vi "Is Command Refnum.vi"(8 "error in (no error)":errorcluster, 11 "Command/Response Refnum in":T1 format="%.0x") -> (0 "error out":errorcluster, 2 "Is Command?":bool, 3 "Command/Response out":string)   [LabVIEW 2018, in "Instrument Addon Scripting API.lvlib"]
uses:
  Instrument Addon Scripting API.lvlib
  <vilib>/NI Veristand/Custom Device API/Custom Device Item Ref.ctl
  Addon/Addon Shared/SubVIs/Constants.vi
  Addon/Addon Shared/Instrument Addon Shared.lvlib
  <vilib>/NI VeriStand/Custom Device API/Custom Device API.lvlib
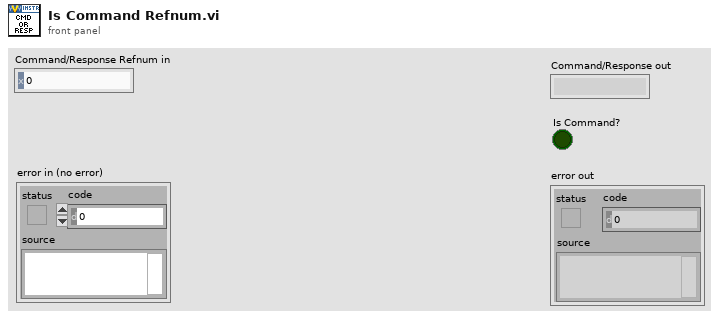
[diagram p1: front panel]
types:
  T1 = typedef "Custom Device API.lvlib/Custom Device Item Ref.ctl" = u64
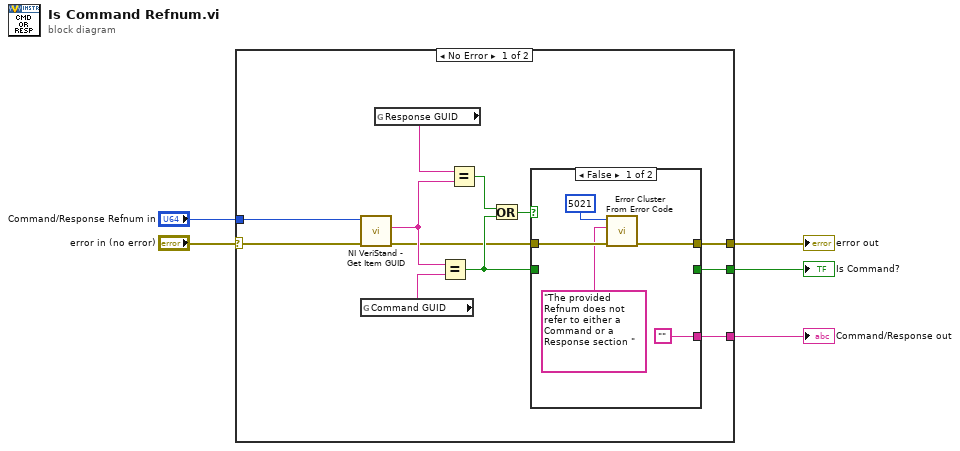
[diagram p0: block diagram]
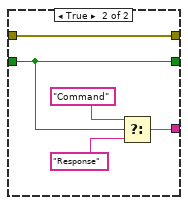
[diagram p2: hidden frame]
diagram:
  n1 = case shown="No Error" "error in (no error)" {
    selector: "error in (no error)" -> [w14 w28]
    tunnel: [w6 _] -> w5
    tunnel: [w8 w28] -> w4
    tunnel: "Command/Response Refnum in" -> [w16 _]
    tunnel: [w15 _] -> w2
    frame No Error {
      n2 = call <vilib>:"NI VeriStand - Get Item GUID.vi"("error in (no error)"=w14, "Item Ref in"=w16) -> ("error out"=w9:errorcluster, "GUID"=w12:string)  [unwired: 7 in, 1 out]
      n3 = global read "Constants.vi" "Command GUID"() -> (w17:string)
      n4 = global read "Constants.vi" "Response GUID"() -> (w13:string)
      n5 = Equal?(x=w12, y=w17) -> (x = y?=w11:bool)
      n6 = Equal?(x=w13, y=w12) -> (x = y?=w10:bool)
      n7 = Or(x=w10, y=w11) -> (x .or. y?=w7:bool)
      n8 = case shown="False" w7 {
        tunnel: ["" w25] -> w15
        tunnel: w11 -> [_ w23]
        tunnel: w9 -> [w21 w24]
        tunnel: [w20 w24] -> w8
        tunnel: [_ w23] -> w6
        frame False {
          n9 = call <vilib>:"Error Cluster From Error Code.vi"("error in (no error)"=w21, "error message (\"\")"="The provided Refnum does not refer to either a Command or a Response section " ("error message (\"\")"), "error code (0)"=5021) -> ("error out"=w20:errorcluster)  [unwired: 6 in]
        }
        frame True {
          n10 = Select(t="Command", s=w23, f="Response") -> (s? t:f=w25:string)
        }
      }
    }
    frame Error {
    }
  }
  "error out" <- w4
  "Command/Response out" <- w2
  "Is Command?" <- w5
